vi "Preview Class Banner Icon.vi"(9 "Banner Color":u32, 10 "Text Color":u32, 11 "Banner Text":string) -> (3 "Class Banner Icon":picture)   [LabVIEW 2015, in "QControl Creation Wizard.lvclass"]
uses:
  QControl Creation Wizard.lvclass
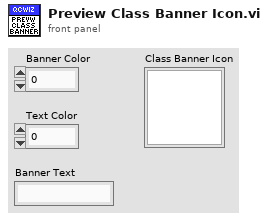
[diagram p1: front panel]
types:
  T1 = enum16{"User-specified Font", "Application Font", "System Font", "Dialog Font"}
  T2 = cluster{"Font Name:":string, "Size":i16, "Strikeout?":bool, "Italic?":bool, "Underline?":bool, "Outline?":bool, "Shadow?":bool, "Bold?":bool}
  T3 = cluster{"horizontal":enum16{"left", "center", "right"}, "vertical":enum16{"top", "center", "bottom"}}
  T4 = cluster{"left":i16, "top":i16, "right":i16, "bottom":i16}
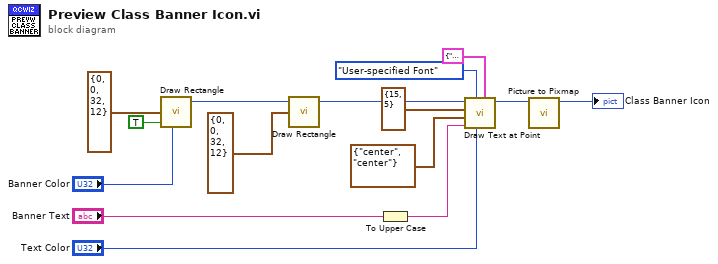
[diagram p0: block diagram]
diagram:
  n1 = call <vilib>:"Draw Rectangle.vi"("rect"=T4 {"left"=0, "top"=0, "right"=32, "bottom"=12}, "fill?(F)"=TRUE, "color(black)"="Banner Color") -> ("new picture"=w4:picture)  [unwired: 6 in]
  n2 = call <vilib>:"Draw Rectangle.vi"("picture"=w4, "rect"=T4 {"left"=0, "top"=0, "right"=32, "bottom"=12}) -> ("new picture"=w6:picture)  [unwired: 7 in]
  n3 = To Upper Case(1:"Banner Text") -> (0:w1:string)
  n4 = call <vilib>:"Draw Text at Point.vi"("[user-specified font]"=T2 {"Font Name:"="Small Fonts", "Size"=8, "Strikeout?"=FALSE, "Italic?"=FALSE, "Underline?"=FALSE, "Outline?"=FALSE, "Shadow?"=FALSE, "Bold?"=FALSE}, "text color(black)"="Text Color", "desired font(Application)"=T1."User-specified Font", "text"=w1, "alignment(left, top)"=T3 {"horizontal"=enum."center", "vertical"=enum."center"}, "origin"=cluster{"x":i16, "y":i16} {"x"=15, "y"=5}, "picture"=w6) -> ("new picture"=w7:picture)  [unwired: 3 in, 1 out]
  n5 = call <vilib>:"Picture to Pixmap.vi"("picture"=w7) -> ("new picture"=→"Class Banner Icon":picture)  [unwired: 9 in, 1 out]
